vi "Encode packed sint64.vi"(7 "Field Number":i32, 10 "sint64":i64[](array[numeric]), 11 "Buffer in":u8[](array[numeric]) format="%.0x") -> (3 "Buffer":u8[](array[numeric]) format="%.0x")   [LabVIEW 2020, in "LV-Proto.lvlib"]
uses:
  LV-Proto.lvlib
  Wire Type.ctl
  Wire Encode Varint I32.vi
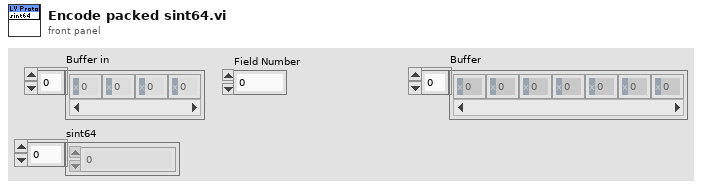
[diagram p1: front panel]
types:
  T1 = typedef "LV-Proto.lvlib/Wire Type.ctl" = enum8{"VARINT", "I64", "LEN", "SGROUP (Deprecated)", "EGROUP (Deprecated)", "I32"}
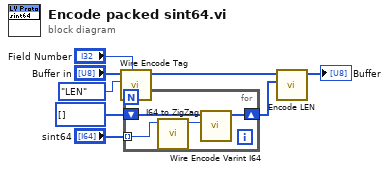
[diagram p0: block diagram]
diagram:
  n1 = call "Wire Encode Tag.vi"("Field Number"="Field Number", "Wire Type"=Wire_Type."LEN", "Buffer in"="Buffer in") -> ("Buffer"=w5:u8[])  [unwired: 8 in]
  n2 = for {
    shift-right: [w12] -> w1
    shift-left: u8[] [] ("Buffer") -> [w9]
    tunnel: "sint64" -> [w11] mode=indexing
    n3 = call "I64 to ZigZag.vi"("sint64"=w11) -> ("ZigZag I64"=w10:i64)  [unwired: 10 in]
    n4 = call "Wire Encode Varint I64.vi"("I64"=w10, "Buffer in"=w9) -> ("Buffer"=w12:u8[])  [unwired: 9 in]
  }
  n5 = call "Encode LEN.vi"("Data"=w1, "Buffer in"=w5) -> ("Buffer"=→"Buffer":u8[])  [unwired: 9 in]
